vi "FGV Automatic Start.vi"(11 "error in (no error)":errorcluster caption="Fehler (Eingang, kein Fehler)", 13 "Aktion":T1) -> (4 "Automaticstart":bool, 15 "error out":errorcluster caption="Fehler (Ausgang)")   [LabVIEW 2020, in "T90.lvlib"]
uses:
  T90.lvlib
  Aktion FGV Automatic Start.ctl
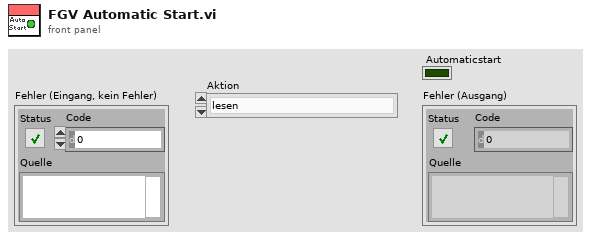
[diagram p1: front panel]
types:
  T1 = typedef "T90.lvlib/Aktion FGV Automatic Start.ctl" = enum16{"lesen", "aktivieren", "deaktivieren"}
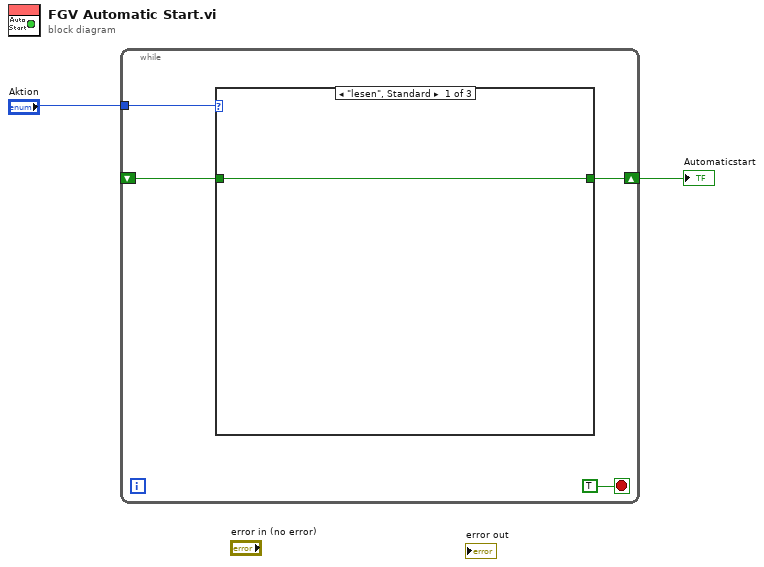
[diagram p0: block diagram]
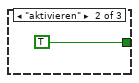
[diagram p2: hidden frame]
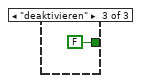
[diagram p3: hidden frame]
diagram:
  n1 = while {
    tunnel: "Aktion" -> [w5]
    shift-right: [w4] -> w2
    shift-left: _ -> [w3]
    stop <- TRUE stop-if-true
    n2 = case shown="\"lesen\", Standard" w5 {
      tunnel: [w7 TRUE FALSE] -> w4
      tunnel: w3 -> [w7 _ _]
      frame "lesen", Default {
      }
      frame "aktivieren" {
      }
      frame "deaktivieren" {
      }
    }
  }
  "Automaticstart" <- w2
